vi "Conversor_float.vi"(2 "subarray":u8[](array[numeric])) -> (5 "Dados":sgl[](array[numeric]))   [LabVIEW 2020]
panel:
  out "sinal":bool
  # "Conversor de dados da serial - quadruplo"
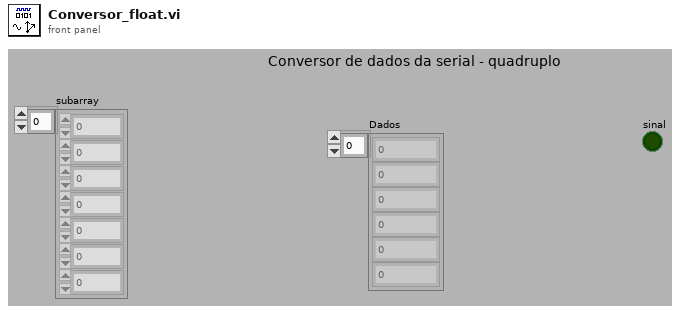
[diagram p1: front panel]
types:
  T1 = cluster{"[0]":u8, "[1]":u8, "[2]":u8, "[3]":u8, "[4]":u8, "[5]":u8, "[6]":u8, "[7]":u8, "[8]":u8}
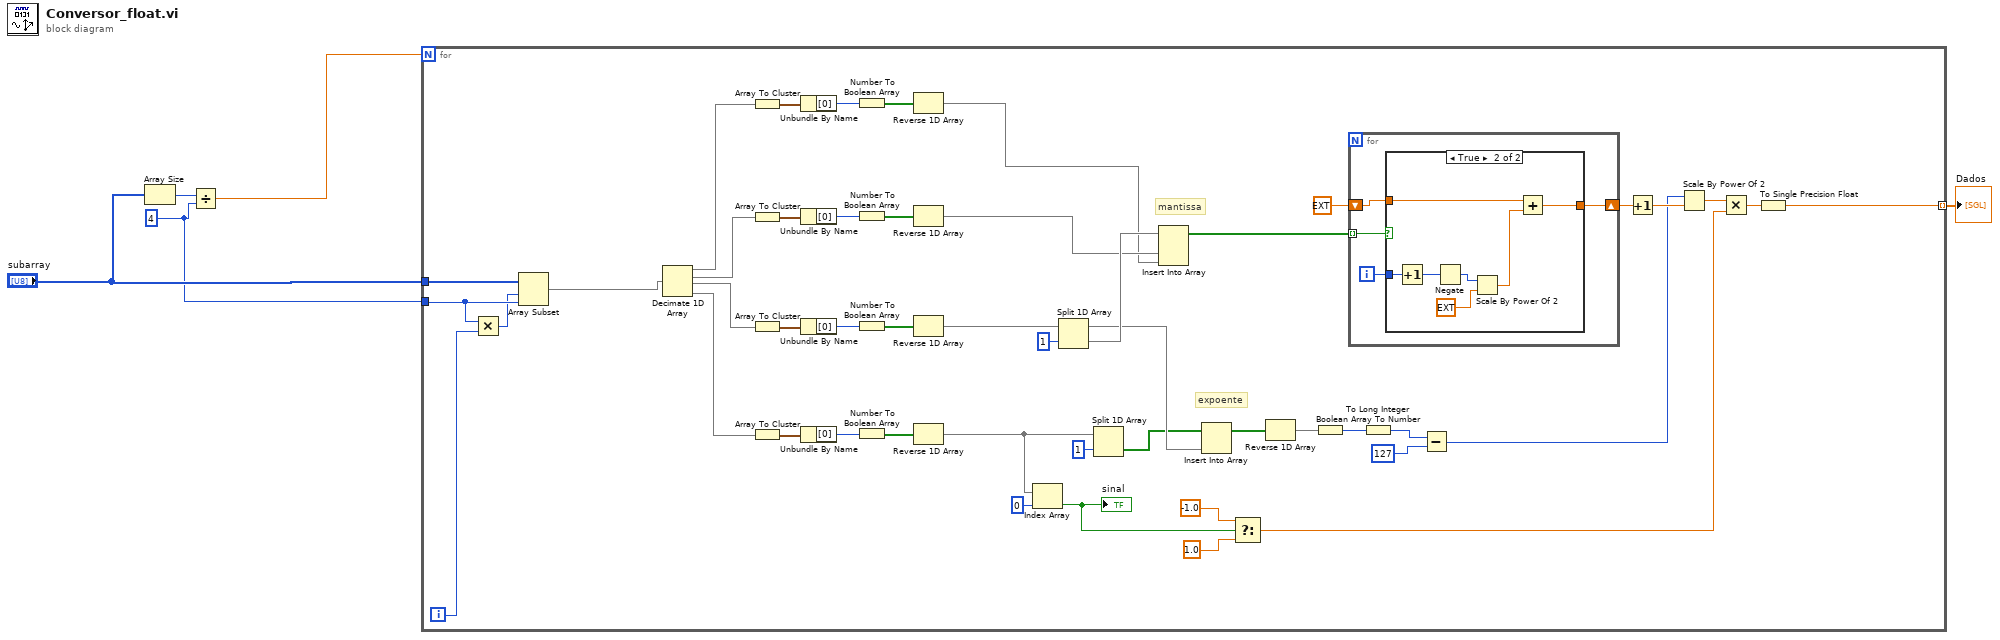
[diagram p0: block diagram]
diagram:
  w1 = 4 ("y")
  n1 = Array Size(array="subarray") -> (size(s)=w5:i32)
  n2 = Divide(x=w5, y=w1) -> (x/y=w4:dbl)
  n3 = for {
    N: w4 -> [_]
    tunnel: "subarray" -> [w10]
    tunnel: [w11] -> w3 mode=indexing
    tunnel: w1 -> [w8]
    i -> [w7]
    # "expoente"
    # "mantissa"
    n4 = Multiply(x=w8, y=w7) -> (x*y=w6:i32)
    n5 = Array Subset(array=w10, index=w6, length=w8) -> (w9:u8[])
    n6 = Decimate 1D Array(w9) -> (w45:u8[], w44:u8[], w43:u8[], w53:u8[])
    n7 = Array To Cluster(array=w45) -> (cluster=w47:T1)
    n8 = Array To Cluster(array=w44) -> (cluster=w49:T1)
    n9 = Array To Cluster(array=w43) -> (cluster=w51:T1)
    n10 = Array To Cluster(array=w53) -> (cluster=w52:T1)
    n11 = Unbundle By Name(w47) -> ("[0]"=w46:u8)
    n12 = Unbundle By Name(w49) -> ("[0]"=w48:u8)
    n13 = Unbundle By Name(w51) -> ("[0]"=w50:u8)
    n14 = Unbundle By Name(w52) -> ("[0]"=w39:u8)
    n15 = Number To Boolean Array(number=w46) -> (Boolean array=w30:bool[])
    n16 = Number To Boolean Array(number=w48) -> (Boolean array=w31:bool[])
    n17 = Number To Boolean Array(number=w50) -> (Boolean array=w32:bool[])
    n18 = Number To Boolean Array(number=w39) -> (Boolean array=w35:bool[])
    n19 = Reverse 1D Array(array=w30) -> (reversed array=w36:bool[])
    n20 = Reverse 1D Array(array=w31) -> (reversed array=w37:bool[])
    n21 = Reverse 1D Array(array=w32) -> (reversed array=w40:bool[])
    n22 = Reverse 1D Array(array=w35) -> (reversed array=w33:bool[])
    n23 = Index Array(array=w33, index=0) -> (element=w22:bool)
    "sinal" <- w22
    n24 = Split 1D Array(array=w40, index=1) -> (first subarray=w15:bool[], second subarray=w38:bool[])
    n25 = Split 1D Array(array=w33, index=1) -> (second subarray=w14:bool[])  [unwired: 1 out]
    n26 = Insert Into Array(array=w38, new element #1=w37, new element #2=w36) -> (w16:bool[])  [unwired: 1 in]
    n27 = Insert Into Array(array=w14, new element=w15) -> (w13:bool[])  [unwired: 1 in]
    n28 = Select(t=-1.0, s=w22, f=1.0) -> (s? t:f=w18:dbl)
    n29 = Reverse 1D Array(array=w13) -> (reversed array=w12:bool[])
    n30 = Boolean Array To Number(Boolean array=w12) -> (number=w26:u32)
    n31 = for {
      tunnel: w16 -> [w57] mode=indexing
      shift-right: [w55] -> w25
      shift-left: ext 0.0 -> [w54]
      i -> [w56]
      n32 = case shown="True" w57 {
        tunnel: w56 -> [_ w65]
        tunnel: [w58 w60] -> w55
        tunnel: w54 -> [w58 w59]
        frame False {
        }
        frame True {
          n33 = Increment(x=w65) -> (x+1=w64:i32)
          n34 = Negate(x=w64) -> (-x=w63:i32)
          n35 = Scale By Power Of 2(n=w63, x=ext 1.0) -> (x*2^n=w61:ext)
          n36 = Add(x=w59, y=w61) -> (x+y=w60:ext)
        }
      }
    }
    n37 = To Long Integer(number=w26) -> (32bit integer=w28:i32)
    n38 = Subtract(x=w28, y=127) -> (x-y=w23:i32)
    n39 = Increment(x=w25) -> (x+1=w24:ext)
    n40 = Scale By Power Of 2(n=w23, x=w24) -> (x*2^n=w19:ext)
    n41 = Multiply(x=w19, y=w18) -> (x*y=w17:ext)
    n42 = To Single Precision Float(number=w17) -> (single precision float=w11:sgl)
  }
  "Dados" <- w3
